vi "Scan Setup.vi"(8 "error in (no error)":errorcluster, 11 "Voltage Pulse Gating System (HV supply) in":refnum<class "Voltage Pulse Gating System (HV supply).lvclass">) -> (0 "error out":errorcluster, 3 "Voltage Pulse Gating System (HV supply) out":refnum<class "Voltage Pulse Gating System (HV supply).lvclass">)   [LabVIEW 2017, in "Voltage Pulse Gating System (HV supply).lvclass"]
doc: "Configure the Instrument based on the class member fields. This step comes after the user has closed the \"Scan Setup\" window and before the actual scan -- so instruments are configured with the user's specified settings."
uses:
  Voltage Pulse Gating System (HV supply).lvclass
  Scanner/Scanner.lvclass
  Instruments/Utility Classes/Scannable/Scannable.lvclass
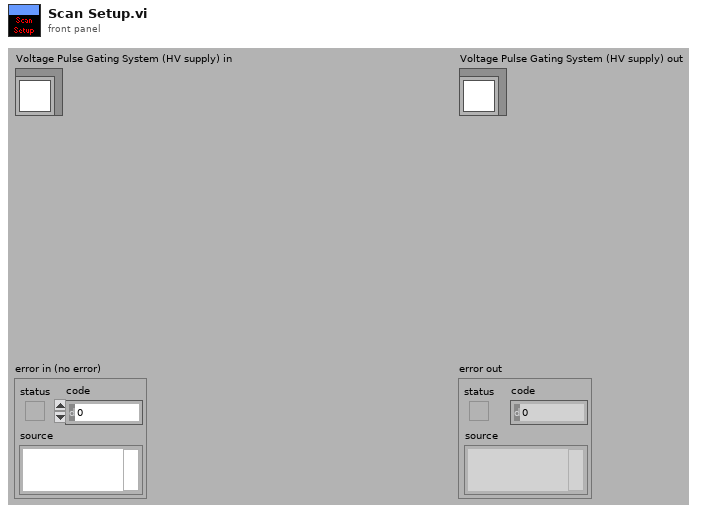
[diagram p1: front panel]
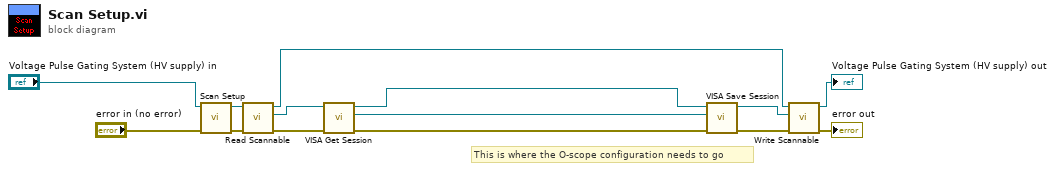
[diagram p0: block diagram]
diagram:
  # "This is where the O-scope configuration needs to go"
  n1 = call-parent "Scan Setup.vi"("error in (no error)"="error in (no error)", "Scanner in"="Voltage Pulse Gating System (HV supply) in") -> ("error out"=w9:errorcluster, "Scanner out"=w12:refnum<class "Voltage Pulse Gating System (HV supply).lvclass">)  [unwired: 8 out]
  n2 = call-dynamic "Read Scannable.vi"("error in (no error)"=w9, "Scanner.lvclass in"=w12) -> ("error out"=w14:errorcluster, "Scannable.lvclass"=w13:refnum<class "Scannable.lvclass">, "Scanner.lvclass out"=w5:refnum<class "Voltage Pulse Gating System (HV supply).lvclass">)  [unwired: 7 out]
  n3 = call-dynamic "VISA Get Session.vi"("error in (no error)"=w14, "Instrument.lvclass in"=w13) -> ("error out"=w8:errorcluster, "VISA Resource Name"=w10:refnum<visa-resource-name>, "Instrument.lvclass out"=w11:refnum<class "Scannable.lvclass">)  [unwired: 7 out]
  n4 = call-dynamic "VISA Save Session.vi"("error in (no error)"=w8, "VISA Resource Name"=w10, "Instrument.lvclass in"=w11) -> ("error out"=w7:errorcluster, "Instrument.lvclass out"=w6:refnum<class "Scannable.lvclass">)  [unwired: 7 out]
  n5 = call-dynamic "Write Scannable.vi"("error in (no error)"=w7, "Scannable.lvclass"=w6, "Scanner.lvclass in"=w5) -> ("error out"=→"error out":errorcluster, "Scanner.lvclass out"=→"Voltage Pulse Gating System (HV supply) out":refnum<class "Voltage Pulse Gating System (HV supply).lvclass">)  [unwired: 7 out]
